vi "Remove Service.vi"(8 "error in (no error)":errorcluster, 10 "Service":refnum<class "Service.lvclass">, 11 "Vecto in":refnum<class "Vecto.lvclass">) -> (0 "error out":errorcluster, 3 "Vecto out":refnum<class "Vecto.lvclass">)   [LabVIEW 2020, in "Vecto.lvlib" / "Vecto.lvclass"]
uses:
  Vecto.lvclass
  Service/Service.lvclass
  Vecto.lvclass/Vecto.ctl
  Service Container/Service Container.lvclass
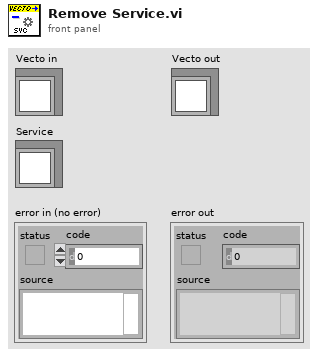
[diagram p1: front panel]
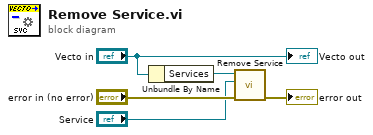
[diagram p0: block diagram]
diagram:
  n1 = Unbundle By Name("Vecto in") -> ("Services"=w5:refnum<class "Service Container.lvclass">)
  n2 = call "Remove Service.vi"("error in (no error)"="error in (no error)", "Service"="Service", "Service Container in"=w5) -> ("error out"=→"error out":errorcluster)  [unwired: 7 in, 1 out]
  "Vecto out" <- "Vecto in"
